vi "模拟量Can应答开关切换.vi"(10 "第几组":u8) -> (0 "超时?":bool, 2 "成功？":bool)   [LabVIEW 2010]
uses:
  全局量/全局_配置.vi
panel:
  in  "匹配CANID":u32 format="%x"
  out "开始时间":dbl format="%#.0f"
  out "接收数据":u8[](array[numeric])
  in  "Baudrate":u32(ring)=1000 caption="K" items=["10"=10, "20"=20, "50"=50, "100"=100, "125"=125, "250"=250, "500"=500, "800"=800, "250"=1000]
  out "Error out":errorcluster {"code" format="%.0x"}
  in  "CANPort":u16
  in  "ReadTimeOut":u32=3000 caption="ms"
  in  "Synchronization":i32(ring)=1 items=["Synchronization"=1, "Asynchronization"=0]
  # "从1开始"
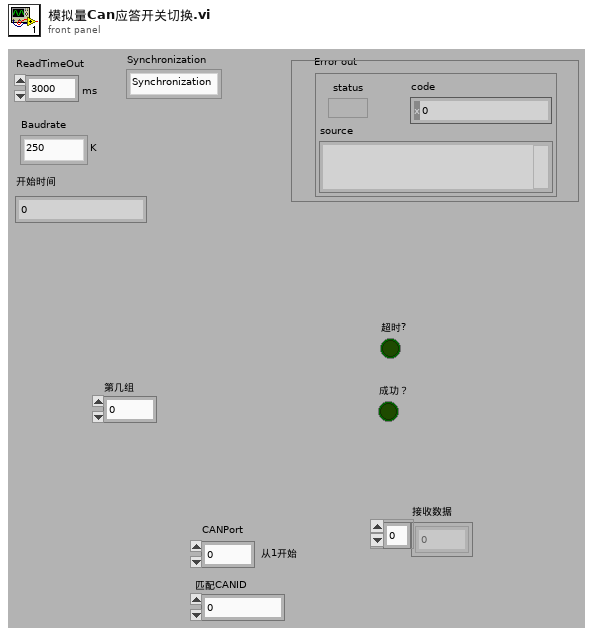
[diagram p1: front panel]
types:
  T1 = cluster{"Internal":u32, "InternalHigh":u32, "Offset":u32, "OffsetHigh":u32, "hEvent":u32}
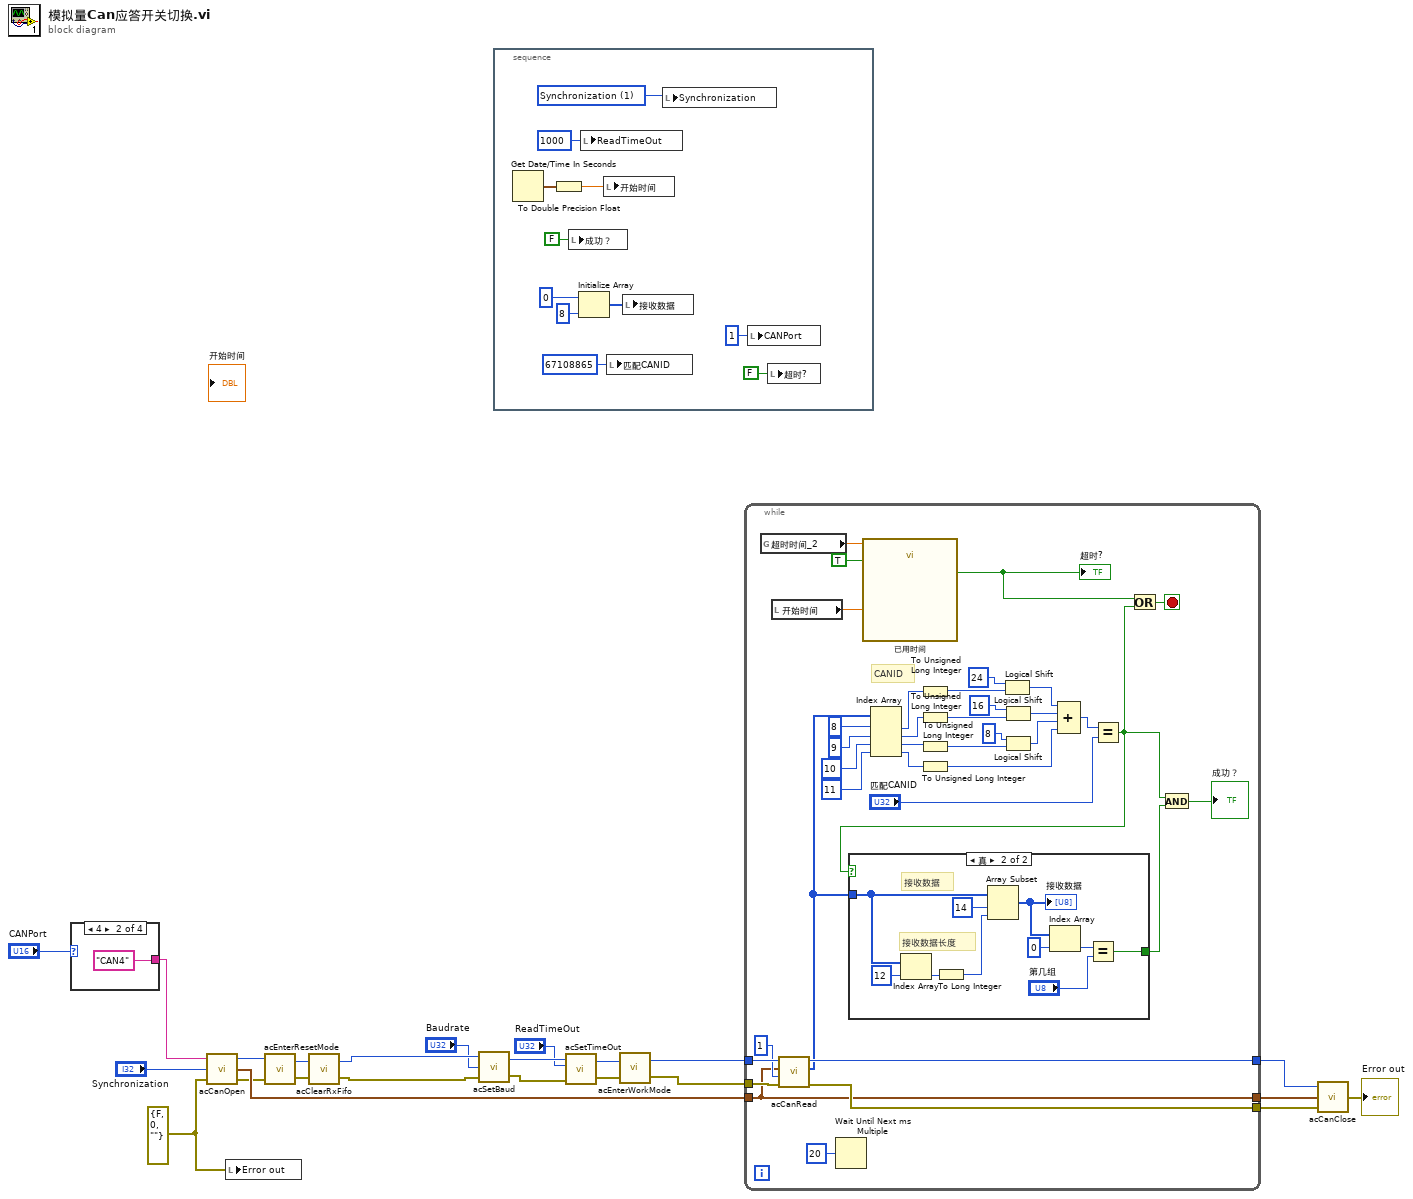
[diagram p0: block diagram]
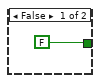
[diagram p2: hidden frame]
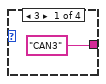
[diagram p3: hidden frame]
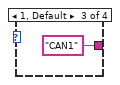
[diagram p4: hidden frame]
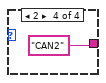
[diagram p5: hidden frame]
diagram:
  w17 = errorcluster {"status"=FALSE, "code"=0, "source"=""} ("Error in")
  n1 = case shown="4" "CANPort" {
    tunnel: ["CAN3" "CAN4" "CAN1" "CAN2"] -> w2
    frame 3 {
    }
    frame 4 {
    }
    frame 1, Default {
    }
    frame 2 {
    }
  }
  n2 = call "acCanOpen.vi"("Error in"=w17, "Synchronization"="Synchronization", "CANPort"=w2) -> ("Error out"=w18:errorcluster, "Overlapped"=w21:T1, "Handle"=w19:u32)
  n3 = local write "Error out"(w17) -> ()
  n4 = call "acEnterResetMode.vi"("Error in"=w18, "Handle  in"=w19) -> ("Error out"=w12:errorcluster, "Handle out"=w11:u32)
  n5 = call "acClearRxFifo.vi"("Error in"=w12, "Handle  in"=w11) -> ("Error out"=w9:errorcluster, "Handle out"=w10:u32)
  n6 = call "acSetBaud.vi"("Error in"=w9, "Baudrate"="Baudrate", "Handle  in"=w10) -> ("Error out"=w14:errorcluster, "Handle out"=w15:u32)
  n7 = stacked-sequence {
    frame #0 {
      w36 = 1 items=["Synchronization"=1, "Asynchronization"=0] ("Synchronization")
      n8 = Get Date/Time In Seconds() -> (seconds since 1Jan1904=w32:timestamp)
      n9 = To Double Precision Float(number=w32) -> (double precision float=w31:dbl)
      n10 = local write "成功？"(FALSE ("成功？")) -> ()
      n11 = Initialize Array(u8 0, 8 ("维数大小")) -> (w33:u8[])
      n12 = local write "ReadTimeOut"(u32 1000 ("ReadTimeOut")) -> ()
      n13 = local write "开始时间"(w31) -> ()
      n14 = local write "匹配CANID"(u32 67108865 ("匹配CANID")) -> ()
      n15 = local write "接收数据"(w33) -> ()
      n16 = local write "Synchronization"(w36) -> ()
      n17 = local write "CANPort"(u16 1 ("CANPort")) -> ()
      n18 = local write "超时?"(FALSE ("超时?")) -> ()
    }
  }
  n19 = call "acSetTimeOut.vi"("Error in"=w14, "Read TimeOut"="ReadTimeOut", "Handle  in"=w15) -> ("Error out"=w7:errorcluster, "Handle out"=w8:u32)  [unwired: 1 in]
  n20 = call "acEnterWorkMode.vi"("Error in"=w7, "Handle  in"=w8) -> ("Error out"=w5:errorcluster, "Handle out"=w6:u32)
  n21 = while {
    tunnel: [w74] -> w22
    tunnel: w21 -> [w69]
    tunnel: [w73] -> w20
    tunnel: w6 -> [w72]
    tunnel: w5 -> [w71]
    tunnel: [w69] -> w1
    stop <- w65 stop-if-true
    # "CANID"
    n22 = global read "全局_配置.vi" "超时时间_2"() -> (w67:dbl)
    n23 = local read "开始时间"() -> (w66:dbl)
    n24 = call "acCanRead.vi"("Error in"=w71, "ReadCount"=u32 1 ("接收CAN帧数 2"), "Overlapped"=w69, "Handle  in"=w72) -> ("Error out"=w73:errorcluster, "MSG"=w43:u8[], "Handle out"=w74:u32)  [unwired: 1 out]
    n25 = Wait Until Next ms Multiple(millisecond multiple=u32 20 ("毫秒倍数")) -> ()  [unwired: 1 out]
    n26 = call "已用时间"("Time Target (s)"=w67, "Reset"=TRUE, "Set Start Time (s)"=w66) -> ("Time has Elapsed"=w39:bool)  [unwired: 9 in, 7 out]
    "超时?" <- w39
    n27 = Index Array(array=w43, index #1=8 ("索引"), index #2=9 ("索引"), index #3=10 ("索引"), index #4=11 ("索引")) -> (element #1=w50:u8, element #2=w49:u8, element #3=w46:u8, element #4=w45:u8)
    n28 = To Unsigned Long Integer(number=w50) -> (unsigned 32bit integer=w51:u32)
    n29 = To Unsigned Long Integer(number=w49) -> (unsigned 32bit integer=w48:u32)
    n30 = To Unsigned Long Integer(number=w46) -> (unsigned 32bit integer=w47:u32)
    n31 = To Unsigned Long Integer(number=w45) -> (unsigned 32bit integer=w44:u32)
    n32 = Logical Shift(y=i8 24, x=w51) -> (x << y=w55:u32)
    n33 = Logical Shift(y=i8 16, x=w48) -> (x << y=w56:u32)
    n34 = Logical Shift(y=i8 8, x=w47) -> (x << y=w54:u32)
    n35 = Compound Arithmetic op=ADD(w55, w56, w54, w44) -> (w53:u32)
    n36 = Equal?(x=w53, y="匹配CANID") -> (x = y?=w42:bool)
    n37 = case shown="真" w42 {
      tunnel: w43 -> [_ w81]
      tunnel: [FALSE w76] -> w41
      frame False {
      }
      frame True {
        # "接收数据"
        # "接收数据长度"
        n38 = Index Array(array=w81, index=12 ("索引")) -> (element=w83:u8)
        n39 = To Long Integer(number=w83) -> (32bit integer=w82:i32)
        n40 = Array Subset(array=w81, index=14 ("索引"), length=w82) -> (w80:u8[])
        "接收数据" <- w80
        n41 = Index Array(array=w80, index=0 ("索引")) -> (element=w78:u8)
        n42 = Equal?(x=w78, y="第几组") -> (x = y?=w76:bool)
      }
    }
    n43 = Or(x=w39, y=w42) -> (x .or. y?=w65:bool)
    n44 = And(x=w42, y=w41) -> (x .and. y?=→"成功？":bool)
  }
  n45 = call "acCanClose.vi"("Error in"=w20, "Overlapped"=w1, "Handle  in"=w22) -> ("Error out"=→"Error out":errorcluster)
